vi "Custom Swerve Drive.vi"(3 "Motor Extremes":T9, 4 "Right Direction Motor Refnum":T2={"DeviceStatus"={"status"=FALSE, "code"=0, "source"=""}, "Type"=enum."PWM", "PWM"={"Digital Module"=enum."Digital Module 1", "PWM Channel"=enum."Invalid", "DeadBand"={"Name"="", "maxPositivePwm"=0, "minPositivePwm"=0, "centerPwm"=0, "maxNegativePwm"=0, "minNegativePwm"=0, "angularRange"=0}}, "CAN"={"Device Number"=0, "Control Mode"=enum."Percent VBus", "Semaphore"=refnum, "Max Vout"=12.0}, "Invert"=FALSE, "TransformRef"=refnum, "InvTransformRef"=refnum}, 5 "Left Direction Motor Refnum":T2={"DeviceStatus"={"status"=FALSE, "code"=0, "source"=""}, "Type"=enum."PWM", "PWM"={"Digital Module"=enum."Digital Module 1", "PWM Channel"=enum."Invalid", "DeadBand"={"Name"="", "maxPositivePwm"=0, "minPositivePwm"=0, "centerPwm"=0, "maxNegativePwm"=0, "minNegativePwm"=0, "angularRange"=0}}, "CAN"={"Device Number"=0, "Control Mode"=enum."Percent VBus", "Semaphore"=refnum, "Max Vout"=12.0}, "Invert"=FALSE, "TransformRef"=refnum, "InvTransformRef"=refnum}, 6 "Robot Drive Refnum":T1={"DevStatus"={"status"=FALSE, "code"=0, "source"=""}, "Motors[]"=[], "Square Inputs"=FALSE, "Max Output"=1.0, "Isochronous"=FALSE}, 7 "Xbox Refnum":T10) -> (1 "Motor Values":dbl[](array[numeric]))   [LabVIEW 2013]
doc: "Utilizes WPI Robotics Library to create a dual-motor swerve drive coupled with an XBox controller."
uses:
  <vilib>/Rock Robotics/WPI/MotorControl/WPI_MotorControlDeviceRef.ctl
  <vilib>/Rock Robotics/SystemInterfaces/Typedef/FPGA_TypedefDigitalModule.ctl
  <vilib>/Rock Robotics/SystemInterfaces/DIO/FPGA_DIOPWMChannel.ctl
  <vilib>/Rock Robotics/WPI/PWM/WPI_PWMDeadband.ctl
  <vilib>/Rock Robotics/WPI/CAN/Jaguar/SubVIs/WPI_CANJaguar_ControlMode.ctl
  <vilib>/Rock Robotics/WPI/PWM/WPI_PWMTransform_ConPane.ctl
  <vilib>/Rock Robotics/WPI/Joystick/WPI_JoystickDevRef.ctl
  <vilib>/Rock Robotics/WPI/Joystick/WPI_JoystickDeviceEnum.ctl
  <vilib>/Rock Robotics/WPI/RobotDrive/WPI_RobotDriveDevRef.ctl
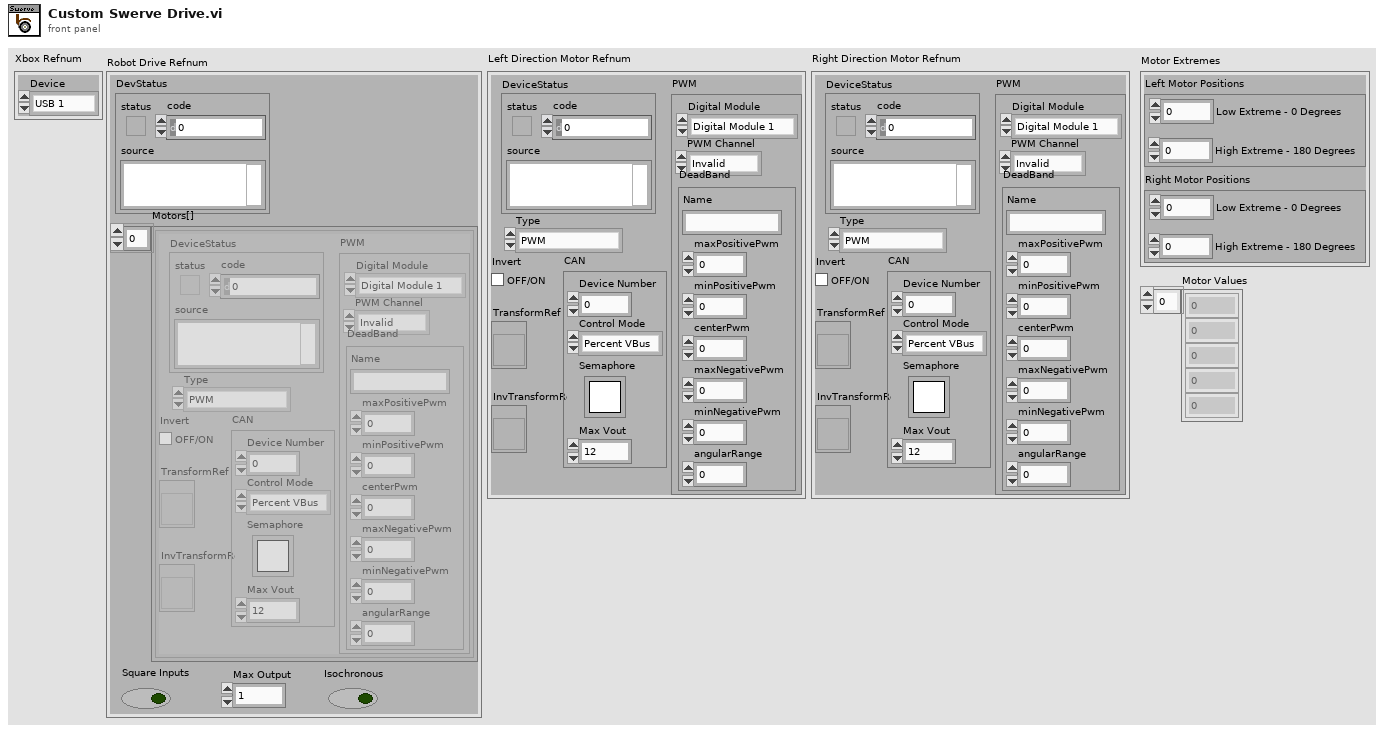
[diagram p1: front panel]
types:
  T1 = typedef "WPI_RobotDriveDevRef.ctl" = cluster{"DevStatus":errorcluster, "Motors[]":T2[], "Square Inputs":bool, "Max Output":dbl, "Isochronous":bool}
  T2 = typedef "WPI_MotorControlDeviceRef.ctl" = cluster{"DeviceStatus":errorcluster, "Type":enum16{"PWM", "CAN"}, "PWM":cluster{"Digital Module":T3, "PWM Channel":T4, "DeadBand":T5}, "CAN":cluster{"Device Number":u8, "Control Mode":T6, "Semaphore":T7, "Max Vout":dbl}, "Invert":bool, "TransformRef":T8, "InvTransformRef":T8}
  T3 = typedef "FPGA_TypedefDigitalModule.ctl" = enum16{"Digital Module 1", "Digital Module 2"}
  T4 = typedef "FPGA_DIOPWMChannel.ctl" = enum8{"PWM 1", "PWM 2", "PWM 3", "PWM 4", "PWM 5", "PWM 6", "PWM 7", "PWM 8", "PWM 9", "PWM 10", "Invalid"}
  T5 = typedef "WPI_PWMDeadband.ctl" = cluster{"Name":string, "maxPositivePwm":i32, "minPositivePwm":i32, "centerPwm":i32, "maxNegativePwm":i32, "minNegativePwm":i32, "angularRange":u16}
  T6 = typedef "WPI_CANJaguar_ControlMode.ctl" = enum8{"Percent VBus", "Current", "Speed", "Position", "Voltage"}
  T7 = typedef "Semaphore RefNum" = refnum<k1>
  T8 = typedef "WPI_PWMTransform_ConPane.ctl" = refnum<vi>
  T9 = cluster{"Left Motor Positions":cluster{"Low Extreme - 0 Degrees":dbl, "High Extreme - 180 Degrees":dbl}, "Right Motor Positions":cluster{"Low Extreme - 0 Degrees":dbl, "High Extreme - 180 Degrees":dbl}}
  T10 = typedef "WPI_JoystickDevRef.ctl" = cluster{"Device":T11}
  T11 = typedef "WPI_JoystickDeviceEnum.ctl" = enum16{"USB 1", "USB 2", "USB 3", "USB 4", "Kinect 1", "Kinect 2"}
  T12 = cluster{"axis 1 (x)":dbl, "axis 2 (y)":dbl, "axis 3 (throttle)":dbl, "axis 4":dbl, "axis 5":dbl, "axis 6":dbl}
  T13 = cluster{"Low Extreme - 0 Degrees":dbl, "High Extreme - 180 Degrees":dbl}
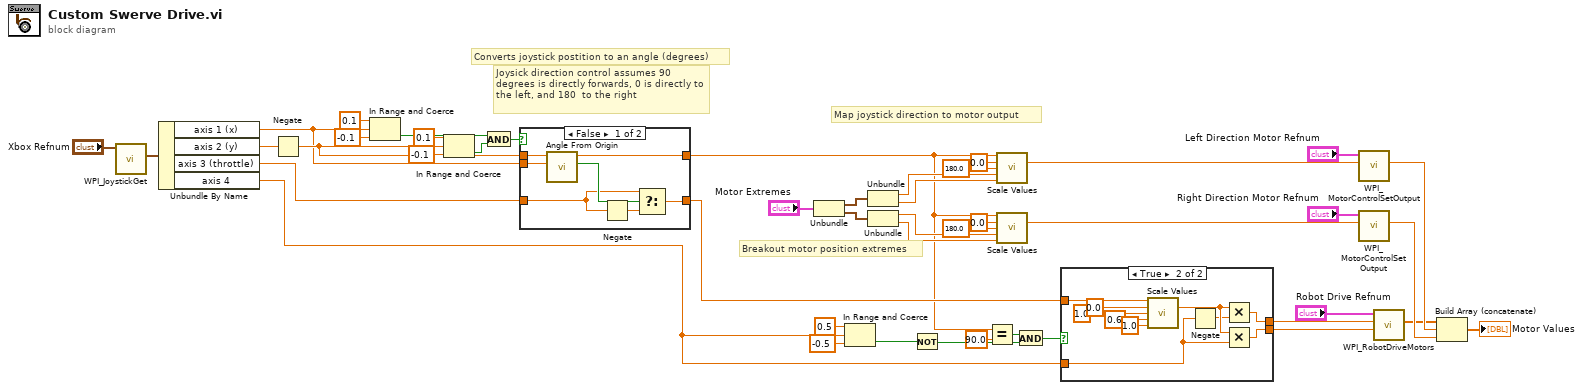
[diagram p0: block diagram]
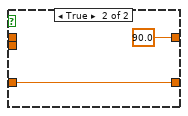
[diagram p2: hidden frame]
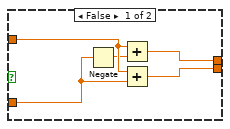
[diagram p3: hidden frame]
diagram:
  # "Joysick direction control assumes 90 degrees is directly forwards, 0 is directly to the left, and 180  to the right"
  # "Breakout motor position extremes"
  # "Converts joystick postition to an angle (degrees)"
  # "Map joystick direction to motor output"
  n1 = call <vilib>:"WPI_JoystickGet.vi"("JoystickDevRef"="Xbox Refnum") -> ("Axes"=w43:T12)  [unwired: 4 in, 2 out]
  n2 = Unbundle By Name(w43) -> ("axis 1 (x)"=w6:dbl, "axis 2 (y)"=w7:dbl, "axis 3 (throttle)"=w5:dbl, "axis 4"=w20:dbl)
  n3 = Negate(x=w7) -> (-x=w8:dbl)
  n4 = In Range and Coerce(upper limit=0.1, x=w6, lower limit=-0.1) -> (In Range?=w10:bool)  [unwired: 1 out]
  n5 = In Range and Coerce(upper limit=0.1, x=w8, lower limit=-0.1) -> (In Range?=w11:bool)  [unwired: 1 out]
  n6 = And(x=w10, y=w11) -> (x .and. y?=w9:bool)
  n7 = case shown="False" w9 {
    tunnel: w6 -> [w48 _]
    tunnel: w8 -> [w49 _]
    tunnel: w5 -> [w46 w54]
    tunnel: [w52 90.0] -> w3
    tunnel: [w51 w54] -> w4
    frame False {
      n8 = call "Angle From Origin.vi"("Y"=w48, "X"=w49) -> ("Above Y Axis?"=w50:bool, "Angle"=w52:dbl)  [unwired: 8 in]
      n9 = Negate(x=w46) -> (-x=w47:dbl)
      n10 = Select(t=w46, s=w50, f=w47) -> (s? t:f=w51:dbl)
    }
    frame True {
    }
  }
  n11 = Unbundle("Motor Extremes") -> ("Left Motor Positions"=w18:T13, "Right Motor Positions"=w17:T13)
  n12 = In Range and Coerce(upper limit=0.5, x=w20, lower limit=-0.5) -> (In Range?=w21:bool)  [unwired: 1 out]
  n13 = Unbundle(w18) -> ("Low Extreme - 0 Degrees"=w38:dbl, "High Extreme - 180 Degrees"=w37:dbl)
  n14 = Unbundle(w17) -> ("Low Extreme - 0 Degrees"=w34:dbl, "High Extreme - 180 Degrees"=w33:dbl)
  n15 = Not(x=w21) -> (.not. x?=w22:bool)
  n16 = Equal?(x=w3, y=90.0) -> (x = y?=w24:bool)
  n17 = call "Scale Values.vi"("input variable"=w3, "input min"=0.0, "input max"=180.0, "output min"=w38, "output max"=w37) -> ("output variable"=w2:dbl)  [unwired: 10 in]
  n18 = call "Scale Values.vi"("input variable"=w3, "input min"=0.0, "input max"=180.0, "output min"=w34, "output max"=w33) -> ("output variable"=w1:dbl)  [unwired: 10 in]
  n19 = And(x=w24, y=w22) -> (x .and. y?=w25:bool)
  n20 = case shown="True" w25 {
    tunnel: w20 -> [w55 w60]
    tunnel: w4 -> [w57 w66]
    tunnel: [w59 w69] -> w27
    tunnel: [w58 w68] -> w26
    frame False {
      n21 = Negate(x=w55) -> (-x=w56:dbl)
      n22 = Add(x=w57, y=w56) -> (x+y=w59:dbl)
      n23 = Add(x=w57, y=w55) -> (x+y=w58:dbl)
    }
    frame True {
      n24 = call "Scale Values.vi"("input variable"=w66, "input min"=0.0, "input max"=1.0, "output min"=0.6, "output max"=1.0) -> ("output variable"=w67:dbl)  [unwired: 10 in]
      n25 = Negate(x=w60) -> (-x=w61:dbl)
      n26 = Multiply(x=w67, y=w61) -> (x*y=w69:dbl)
      n27 = Multiply(x=w67, y=w60) -> (x*y=w68:dbl)
    }
  }
  n28 = call <vilib>:"WPI_MotorControlSetOutput.vi"("Output"=w2, "MotorControlDevRef"="Left Direction Motor Refnum") -> ("Motor Output"=w32:dbl)  [unwired: 7 in, 2 out]
  n29 = call <vilib>:"WPI_MotorControlSetOutput.vi"("Output"=w1, "MotorControlDevRef"="Right Direction Motor Refnum") -> ("Motor Output"=w31:dbl)  [unwired: 7 in, 2 out]
  n30 = call <vilib>:"WPI_RobotDriveMotors.vi"("RightSpeed"=w26, "LeftSpeed"=w27, "RobotDriveDevRef"="Robot Drive Refnum") -> ("Motor Values"=w30:dbl[])  [unwired: 6 in, 2 out]
  n31 = Build Array (concatenate)(w30, w32, w31) -> (→"Motor Values":dbl[])
